vi "Set Cell Value.vi"(7 "Sheet Name":string, 8 "error in":errorcluster, 9 "Value":string, 10 "Cell Address":string, 11 "SpreadsheetDocument":refnum<k24>) -> (0 "error out":errorcluster, 3 "SpreadsheetDocument out":refnum<k24>)   [LabVIEW 2021, in "Open Xml.lvlib"]
uses:
  Open Xml.lvlib
  D:/git/Open-Xml-LabVIEW/dll/DocumentFormat.OpenXml.dll
  dll/DocumentFormat.OpenXml.dll
  D:/git/Open-Xml-LabVIEW/dll/OpenXmlGenericsWrapper.dll
  dll/OpenXmlGenericsWrapper.dll
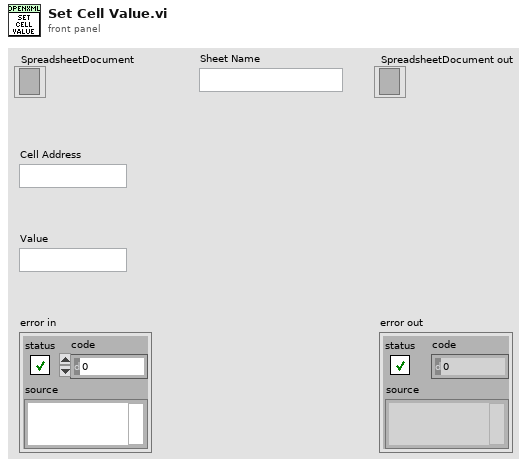
[diagram p1: front panel]
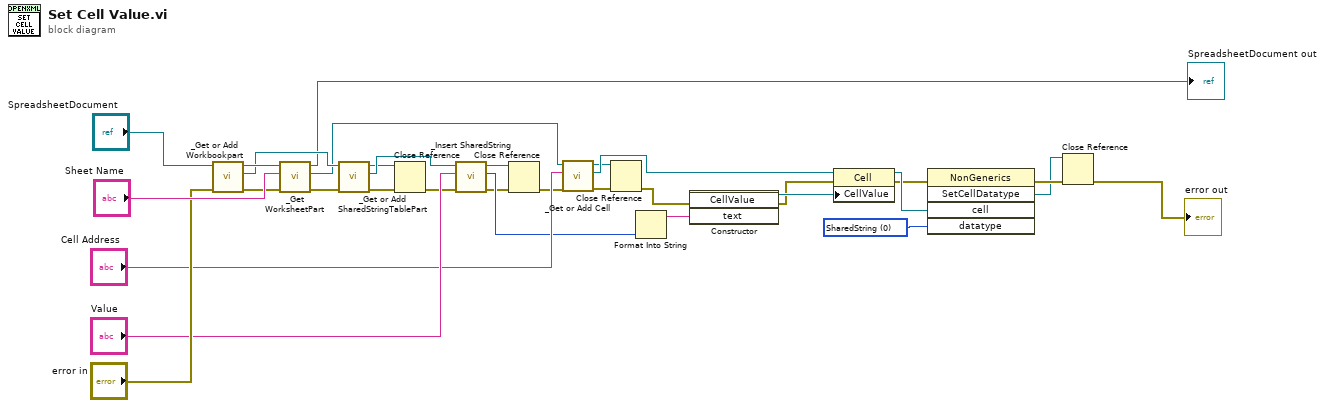
[diagram p0: block diagram]
diagram:
  w10 = 0 items=["SharedString"] ("datatype")
  n1 = call "_Get or Add Workbookpart.vi"("error in"="error in", "SpreadsheetDocument"="SpreadsheetDocument") -> ("error out"=w28:errorcluster, "WorkbookPart"=w25:refnum<k24>, "SpreadsheetDocument out"=w29:refnum<k24>)  [unwired: 7 in]
  n2 = call "_Get WorksheetPart.vi"("error in"=w28, "Sheet Name"="Sheet Name", "SpreadsheetDocument in"=w29) -> ("error out"=w27:errorcluster, "WorksheetPart"=w20:refnum<k24>, "SpreadsheetDocument out"=→"SpreadsheetDocument out":refnum<k24>)  [unwired: 6 in]
  n3 = call "_Get or Add SharedStringTablePart.vi"("error in"=w27, "WorkbookPart"=w25) -> ("error out"=w26:errorcluster, "SharedStringTablePart"=w24:refnum<k24>, "WorkbookPart"=w21:refnum<k24>)  [unwired: 7 in]
  n4 = Close Reference(reference=w21, error in (no error)=w26) -> (error out=w22:errorcluster)
  n5 = call "_Insert SharedString.vi"("error in"=w22, "Value"="Value", "SharedStringTablePart in"=w24) -> ("error out"=w1:errorcluster, "Index"=w4:i32, "SharedStringTablePart out"=w2:refnum<k24>)  [unwired: 6 in]
  n6 = Close Reference(reference=w2, error in (no error)=w1) -> (error out=w3:errorcluster)
  n7 = call "_Get or Add Cell.vi"("error in"=w3, "Cell Address"="Cell Address", "Worksheetpart in"=w20) -> ("error out"=w13:errorcluster, "Cell"=w18:refnum<k24>, "WorksheetPart out"=w5:refnum<k24>)  [unwired: 6 in]
  n8 = Close Reference(reference=w5, error in (no error)=w13) -> (error out=w6:errorcluster)
  n9 = Format Into String(w4) -> (resulting string=w17:string)  [unwired: 3 in, 1 out]
  n10 = constructor class="CellValue"(error in=w6, "text"=w17) -> (reference out=w16:refnum<k24>, error out=w12:errorcluster)  [unwired: 2 in, 2 out]
  n11 = property class="Cell"(reference=w18, error in=w12, "CellValue"=w16) -> (reference out=w11:refnum<k24>, error out=w9:errorcluster)
  n12 = invoke class="NonGenerics" method="SetCellDatatype"(error in=w9, "cell"=w11, "datatype"=w10) -> (error out=w8:errorcluster, "SetCellDatatype"=w7:refnum<k24>)  [unwired: 2 in, 3 out]
  n13 = Close Reference(reference=w7, error in (no error)=w8) -> (error out=→"error out":errorcluster)
